vi "Init 2 Talon Drive Motors With CVS Files.vi"(2 "error in":errorcluster, 3 "Robot ID":string="985") -> (0 "error out":errorcluster, 1 "RobotDriveDevRef":T1)   [LabVIEW 2019]
uses:
  <vilib>/Rock Robotics/WPI/RobotDrive/WPI_RobotDriveDevRef.ctl
  <vilib>/Rock Robotics/WPI/MotorControl/WPI_MotorControlDeviceRef.ctl
  <vilib>/Rock Robotics/WPI/MotorControl/WPI_MotorControlType.ctl
  <vilib>/Rock Robotics/SystemInterfaces/DIO/FPGA_DIOPWMChannel.ctl
  <vilib>/Rock Robotics/WPI/PWM/WPI_PWMDeadband.ctl
  <vilib>/Rock Robotics/SystemInterfaces/DIO/FPGA_DIOChannel.ctl
  <vilib>/Rock Robotics/WPI/SafetyOutput/WPI_SafetyOutputConfigMenu.ctl
  <vilib>/Rock Robotics/WPI/RobotDrive/WPI_RobotDriveOpen2MotorWithExistingMotors.vi
  <vilib>/Rock Robotics/WPI/RobotDrive/WPI_RobotDriveOpen2MotorWithTalon.vi
panel:
  out "Drive Right Front":u8
  out "Drive Left Front":u8
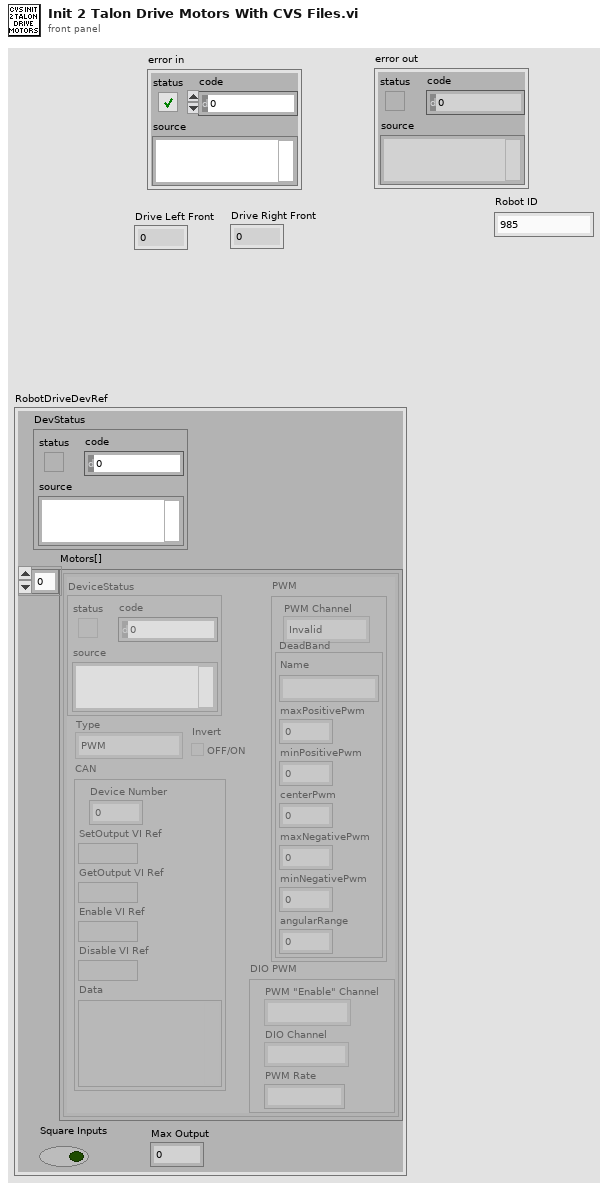
[diagram p1: front panel]
types:
  T1 = typedef "WPI_RobotDriveDevRef.ctl" = cluster{"DevStatus":errorcluster, "Motors[]":T2[], "Square Inputs":bool, "Max Output":dbl}
  T2 = typedef "WPI_MotorControlDeviceRef.ctl" = cluster{"DeviceStatus":errorcluster, "Type":T3, "PWM":cluster{"PWM Channel":T4, "DeadBand":T5}, "CAN":cluster{"Device Number":u8, "SetOutput VI Ref":variant, "GetOutput VI Ref":variant, "Enable VI Ref":variant, "Disable VI Ref":variant, "Data":variant}, "Invert":bool, "DIO PWM":cluster{"PWM \"Enable\" Channel":T4, "DIOChannel":T6, "PWM Rate":dbl}}
  T3 = typedef "WPI_MotorControlType.ctl" = enum16{"PWM", "CAN", "DIO PWM"}
  T4 = typedef "FPGA_DIOPWMChannel.ctl" = enum8{"PWM 0", "PWM 1", "PWM 2", "PWM 3", "PWM 4", "PWM 5", "PWM 6", "PWM 7", "PWM 8", "PWM 9", "PWM MXP 0", "PWM MXP 1", "PWM MXP 2", "PWM MXP 3", "PWM MXP 4", "PWM MXP 5", "PWM MXP 6", "PWM MXP 7", "PWM MXP 8", "PWM MXP 9", "Invalid"}
  T5 = typedef "WPI_PWMDeadband.ctl" = cluster{"Name":string, "maxPositivePwm":i32, "minPositivePwm":i32, "centerPwm":i32, "maxNegativePwm":i32, "minNegativePwm":i32, "angularRange":u16}
  T6 = typedef "FPGA_DIOChannel.ctl" = enum8{"DIO 0", "DIO 1", "DIO 2", "DIO 3", "DIO 4", "DIO 5", "DIO 6", "DIO 7", "DIO 8", "DIO 9", "DIO MXP 0", "DIO MXP 1", "DIO MXP 2", "DIO MXP 3", "DIO MXP 4", "DIO MXP 5", "DIO MXP 6", "DIO MXP 7", "DIO MXP 8", "DIO MXP 9", "DIO MXP 10", "DIO MXP 11", "DIO MXP 12", "DIO MXP 13", "DIO MXP 14", "DIO MXP 15", "SPI Port CS1", "SPI Port CS2", "SPI Port CS3", "SPI Port MISO", "SPI Port MOSI", "Invalid"}
  T7 = typedef "WPI_SafetyOutputConfigMenu.ctl" = enum16{"Enable", "Disable"}
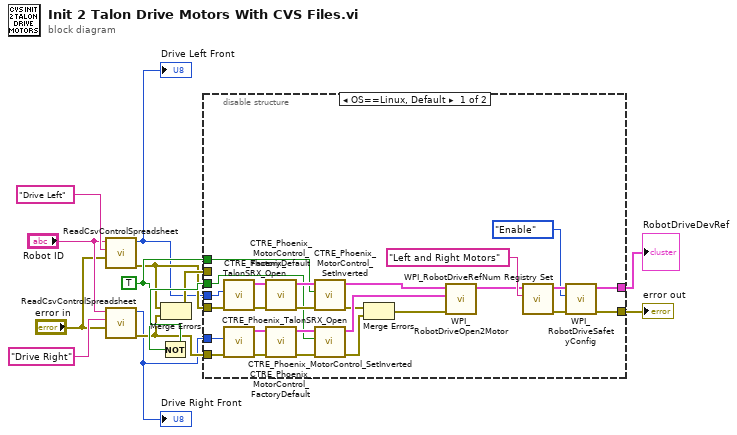
[diagram p0: block diagram]
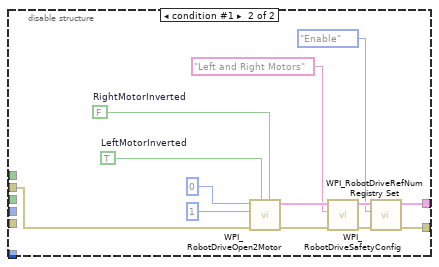
[diagram p2: hidden frame]
diagram:
  w10 = TRUE ("Invert")
  n1 = call "ReadCsvControlSpreadsheet.vi"("error in"="error in", "Motor ID"="Drive Left", "Robot ID"="Robot ID") -> ("error out"=w5:errorcluster, "Can Bus ID"=w2:u8)  [unwired: 7 out]
  "Drive Left Front" <- w2
  n2 = call "ReadCsvControlSpreadsheet.vi"("error in"="error in", "Motor ID"="Drive Right", "Robot ID"="Robot ID") -> ("error out"=w4:errorcluster, "Can Bus ID"=w1:u8)  [unwired: 7 out]
  "Drive Right Front" <- w1
  n3 = Not(x=w10) -> (.not. x?=w11:bool)
  n4 = Merge Errors(w5, w4) -> (w7:errorcluster)
  n5 = disable-structure shown="OS==Linux, Default" {
    disable-tunnel: w11 -> [w14 _]
    disable-tunnel: w10 -> [w17 _]
    disable-tunnel: w2 -> [w19 _]
    disable-tunnel: w1 -> [w16 _]
    disable-tunnel: [w35 w43] -> w8
    disable-tunnel: w7 -> [_ w42]
    disable-tunnel: [w32 w40] -> w6
    disable-tunnel: w5 -> [w18 _]
    disable-tunnel: w4 -> [w15 _]
    frame condition #0 (active) {
      n6 = call <vilib>:"CTRE_Phoenix_TalonSRX_Open.vi"("error in"=w18, "Device Number"=w19) -> ("error out"=w28:errorcluster, "CAN Talon SRX Ref"=w29:T2)  [unwired: 8 in]
      n7 = call <vilib>:"CTRE_Phoenix_TalonSRX_Open.vi"("error in"=w15, "Device Number"=w16) -> ("error out"=w23:errorcluster, "CAN Talon SRX Ref"=w24:T2)  [unwired: 8 in]
      n8 = call <vilib>:"CTRE_Phoenix_MotorControl_FactoryDefault.vi"("error in"=w28, "PhoenixMotorControlDevRef"=w29) -> ("error out"=w30:errorcluster, "PhoenixMotorControlDevRef"=w31:T2)  [unwired: 8 in]
      n9 = call <vilib>:"CTRE_Phoenix_MotorControl_FactoryDefault.vi"("error in"=w23, "PhoenixMotorControlDevRef"=w24) -> ("error out"=w25:errorcluster, "PhoenixMotorControlDevRef"=w26:T2)  [unwired: 8 in]
      n10 = call <vilib>:"CTRE_Phoenix_MotorControl_SetInverted.vi"("error in (no error)"=w30, "Invert?"=w17, "PhoenixMotorControlDevRef"=w31) -> ("error out"=w21:errorcluster, "PhoenixMotorControlDevRef"=w27:T2)  [unwired: 7 in]
      n11 = call <vilib>:"CTRE_Phoenix_MotorControl_SetInverted.vi"("error in (no error)"=w25, "Invert?"=w14, "PhoenixMotorControlDevRef"=w26) -> ("error out"=w20:errorcluster, "PhoenixMotorControlDevRef"=w22:T2)  [unwired: 7 in]
      n12 = Merge Errors(w21, w20) -> (w34:errorcluster)
      n13 = call-poly <vilib>:"WPI_RobotDriveOpen2Motor.vi"("error in (no error)"=w34, "Right Motor Dev Ref"=w22, "Left Motor Dev Ref"=w27) -> ("RobotDriveDevRef"=w36:T1)  [unwired: 7 in, 1 out]
      n14 = call <vilib>:"WPI_RobotDriveRefNum Registry Set.vi"("refnum name"="Left and Right Motors", "RobotDriveDevRef"=w36) -> ("error out"=w33:errorcluster, "RobotDriveDevRef"=w39:T1)  [unwired: 2 in, 6 out]
      n15 = call <vilib>:"WPI_RobotDriveSafetyConfig.vi"("error in (no error)"=w33, "mode"=WPI_SafetyOutputConfigMenu."Enable", "RobotDriveDevRef"=w39) -> ("error out"=w32:errorcluster, "RobotDriveDevRef"=w35:T1)  [unwired: 7 in]
    }
    frame condition #1 {
      w47 = TRUE  # LeftMotorInverted
      w48 = FALSE  # RightMotorInverted
      n16 = call-poly <vilib>:"WPI_RobotDriveOpen2Motor.vi"("Right Motor Inverted"=w48, "Left Motor Inverted"=w47, "error in (no error)"=w42, "Right Motor"=u8 1 ("Left Motor"), "Left Motor"=u8 0) -> ("error out"=w51:errorcluster, "RobotDriveDevRef"=w50:T1)  [unwired: 5 out]
      n17 = call <vilib>:"WPI_RobotDriveRefNum Registry Set.vi"("error in (no error)"=w51, "refnum name"="Left and Right Motors", "RobotDriveDevRef"=w50) -> ("error out"=w41:errorcluster, "RobotDriveDevRef"=w52:T1)  [unwired: 1 in, 6 out]
      n18 = call <vilib>:"WPI_RobotDriveSafetyConfig.vi"("error in (no error)"=w41, "mode"=WPI_SafetyOutputConfigMenu."Enable", "RobotDriveDevRef"=w52) -> ("error out"=w40:errorcluster, "RobotDriveDevRef"=w43:T1)  [unwired: 7 in]
    }
  }
  "RobotDriveDevRef" <- w8
  "error out" <- w6
